vi "Calibration Utility.vi"() -> ()   [LabVIEW 2019]
panel:
  in  "Tab 1":enum32{"Page 1", "Page 2"}(tab)
  in  "Main Tab":T1(tab)
  in  "Tab 2":enum32{"Page 1", "Page 2"}(tab)
  out "Title":string="Calibration Utility, vBETA1"
  out "Date":string="2/21/2012"
  out "Time":string="2:11:48 PM"
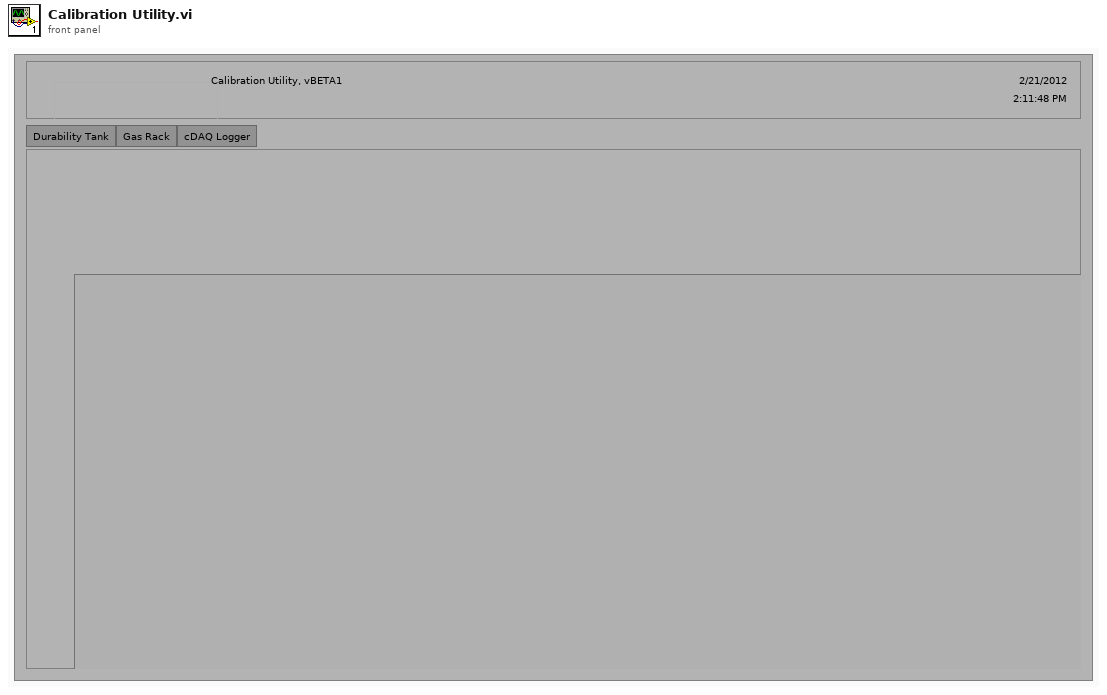
[diagram p1: front panel]
types:
  T1 = enum32{"Netway", "Durability Tank", "Gas Rack", "cDAQ Logger", "Dunk Tank"}
  T2 = cluster{"Error":errorcluster, "OldTab":enum32{"Netway", "Durability Tank", "Gas Rack", "cDAQ Logger", "Dunk Tank"}}
  T3 = enum32{"Page Enabled", "Page Disabled", "Page Disabled & Grayed"}
  T4 = enum32{"Invalid", "Standard", "Closed", "Hidden", "Minimized", "Maximized"}
  T5 = enum32{"invalid app kind", "Development System", "Run Time System", "Student Edition", "Embedded LabVIEW", "Evaluation", "Custom"}
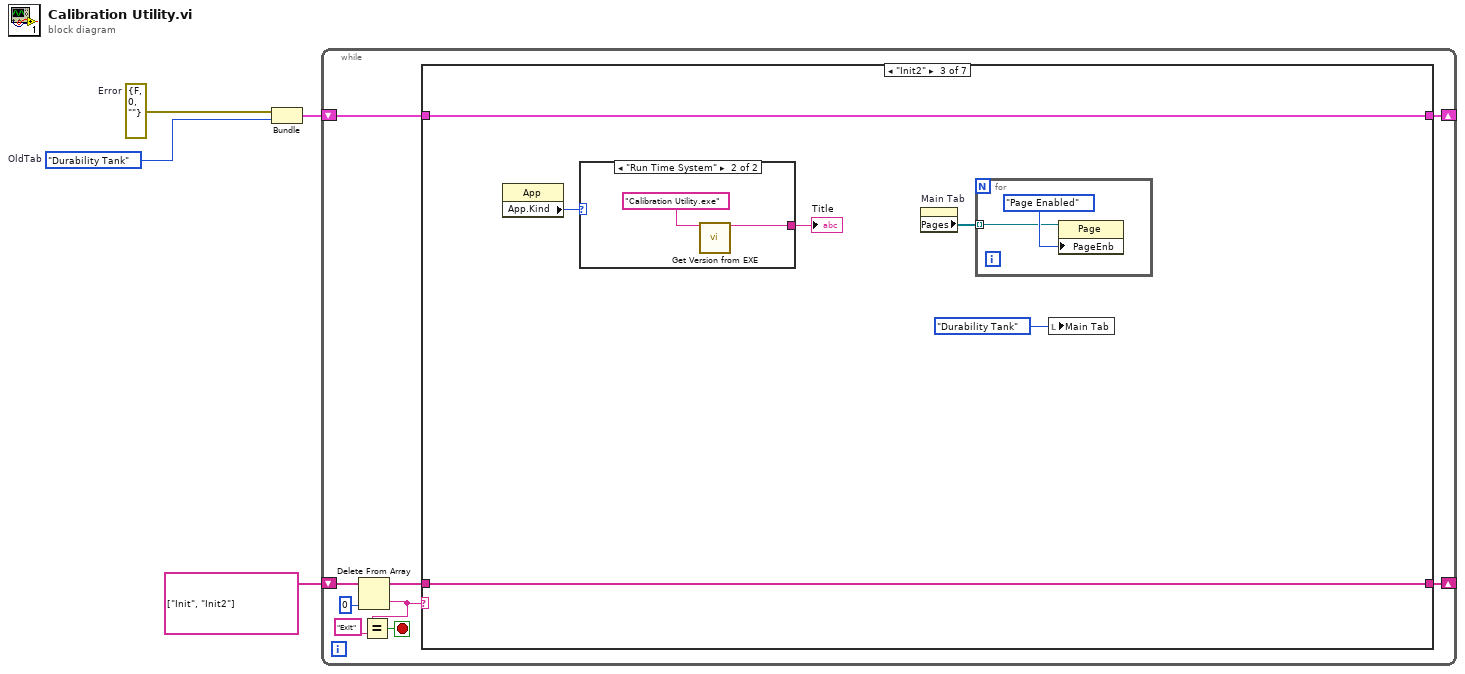
[diagram p0: block diagram]
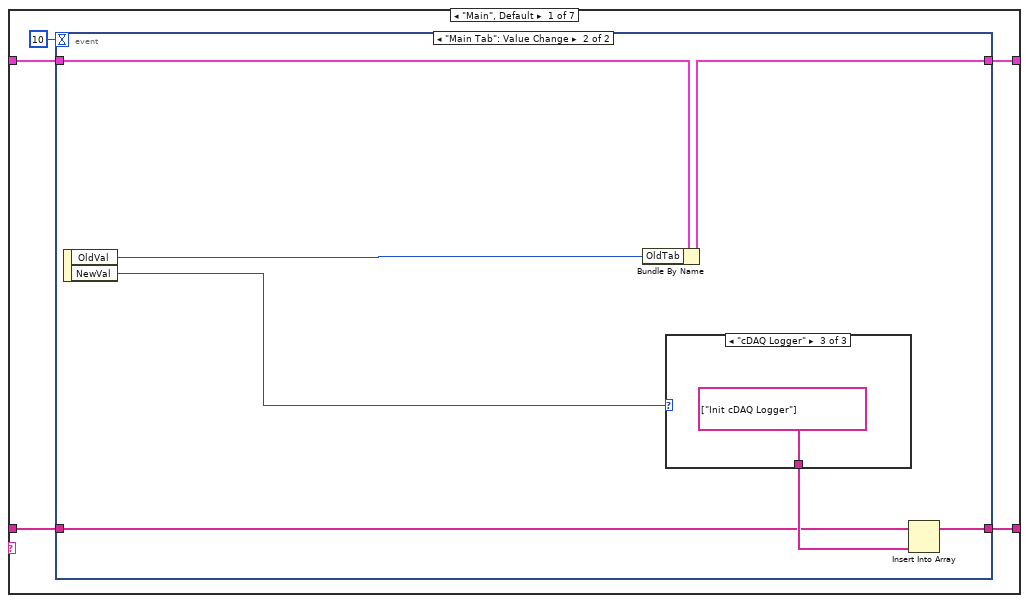
[diagram p2: hidden frame]
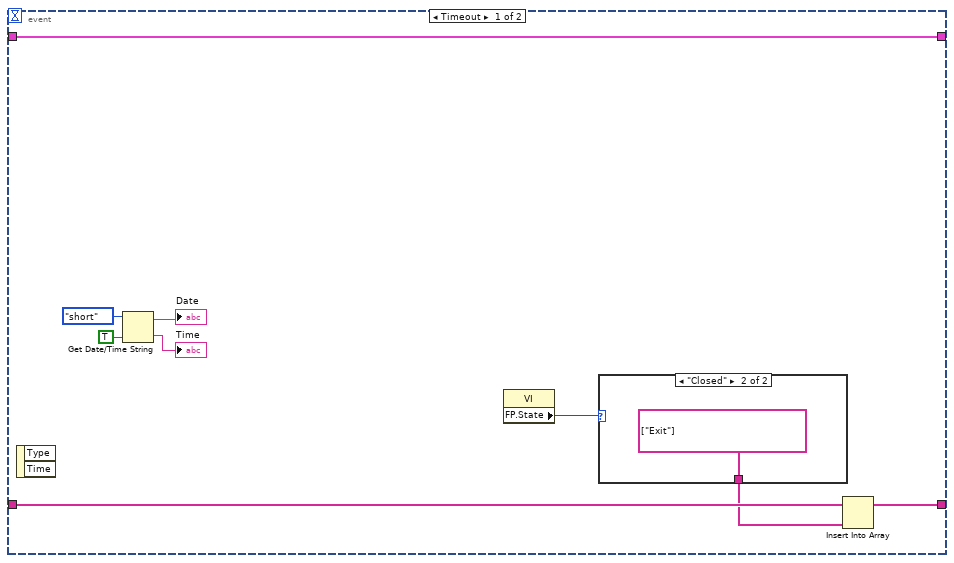
[diagram p3: hidden frame]
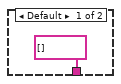
[diagram p4: hidden frame]
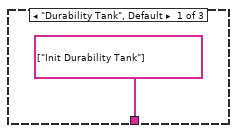
[diagram p5: hidden frame]
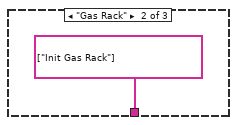
[diagram p6: hidden frame]
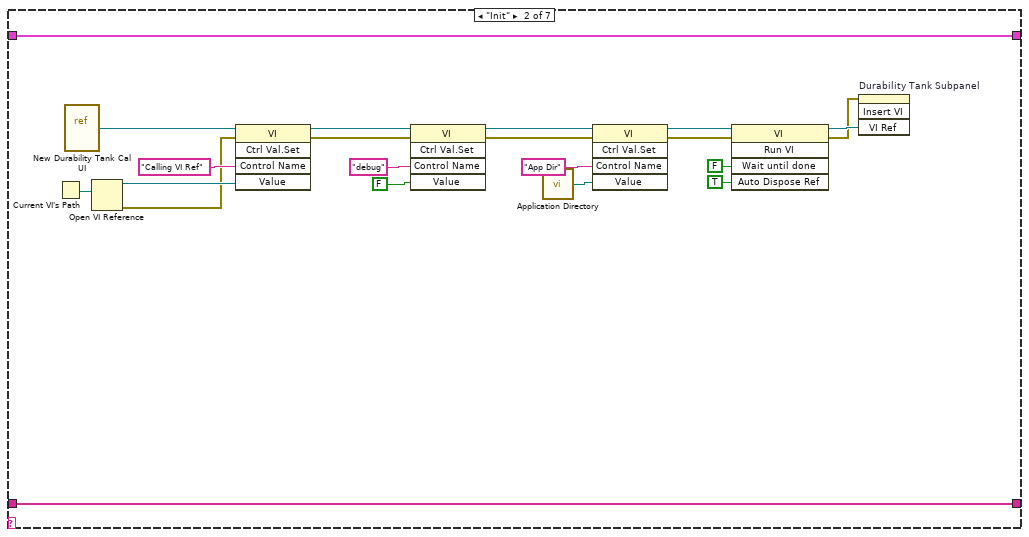
[diagram p7: hidden frame]
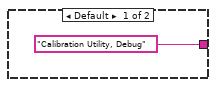
[diagram p8: hidden frame]
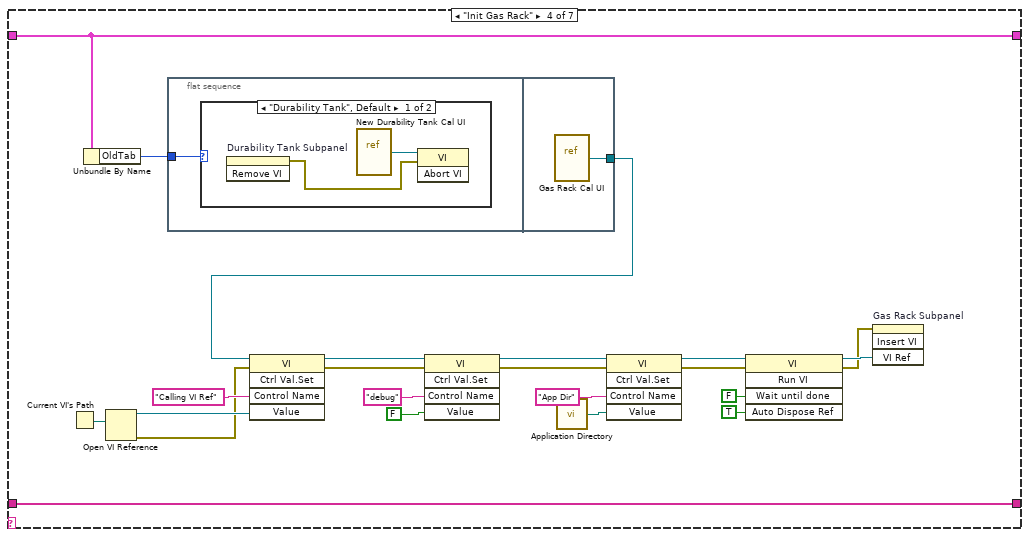
[diagram p9: hidden frame]
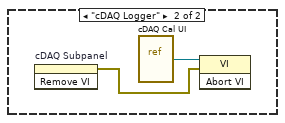
[diagram p10: hidden frame]
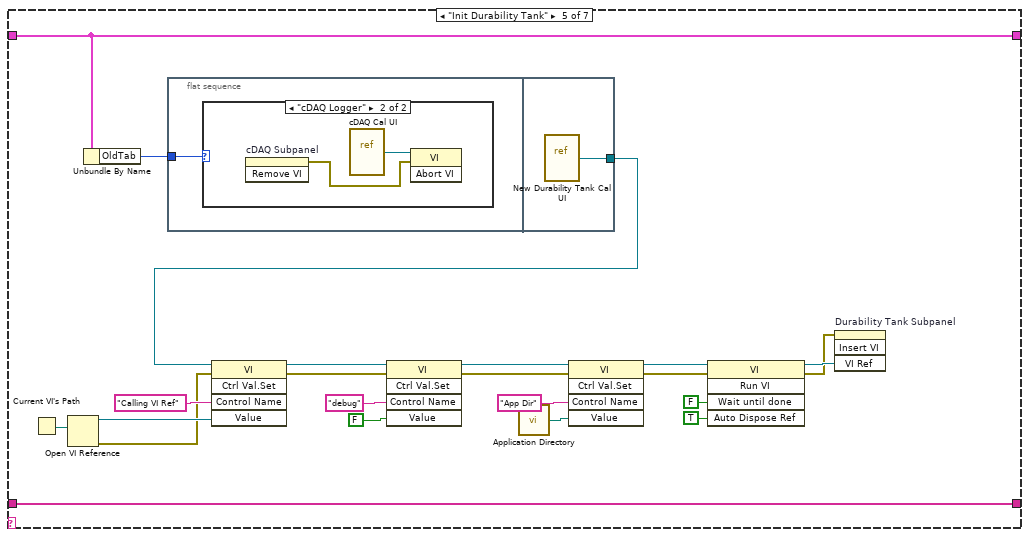
[diagram p11: hidden frame]
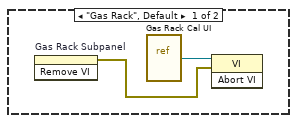
[diagram p12: hidden frame]
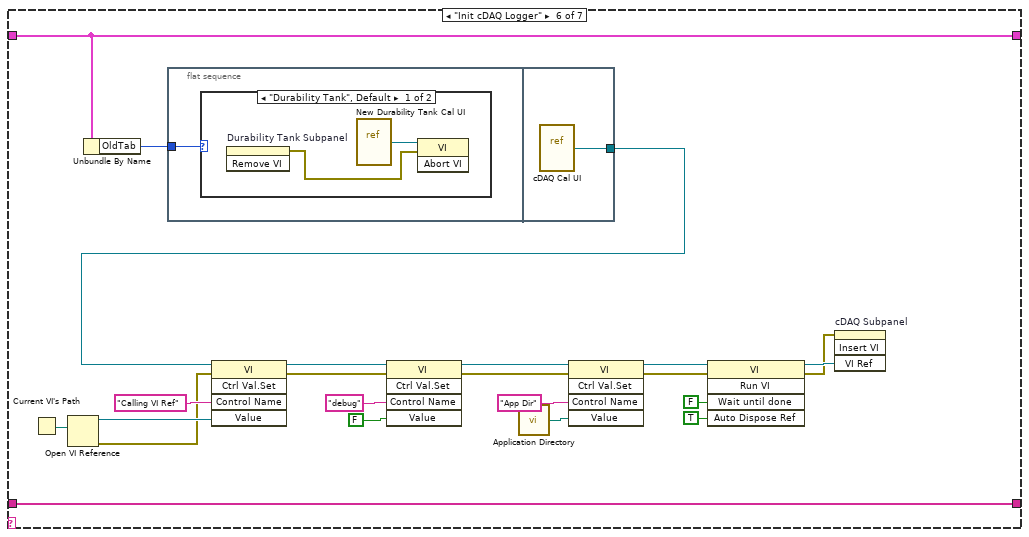
[diagram p13: hidden frame]
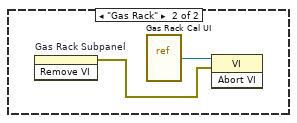
[diagram p14: hidden frame]
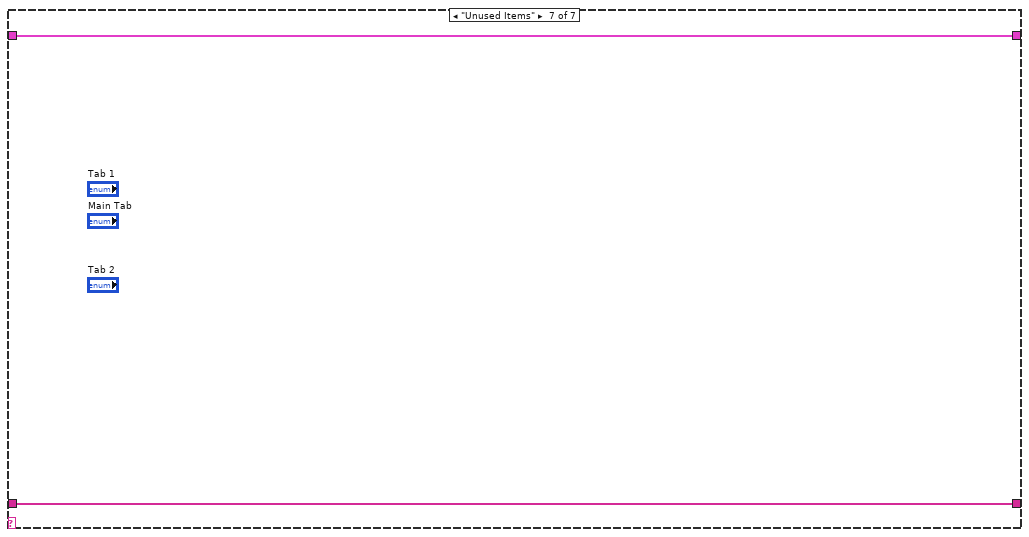
[diagram p15: hidden frame]
diagram:
  w1 = T1."Durability Tank"  # OldTab
  w2 = errorcluster {"status"=FALSE, "code"=0, "source"=""}  # Error
  n1 = Bundle("Error"=w2, "OldTab"=w1) -> (w3:T2)  [unwired: 1 in]
  n2 = while {
    shift-right: [w10] -> _
    shift-left: string[] ["Init", "Init2"] -> [w13]
    shift-right: [w6] -> _
    shift-left: w3 -> [w7]
    stop <- w12 stop-if-true
    n3 = Delete From Array(array=w13, index=0) -> (deleted portion=w9:string, array with subset deleted=w11:string[])  [unwired: 1 in]
    n4 = Equal?(x=w9, y="Exit" ("x")) -> (x = y?=w12:bool)
    n5 = case shown="\"Init2\"" w9 {
      tunnel: [w16 w60 w65 w93 w121 w149 w156] -> w10
      tunnel: w11 -> [w17 w60 w65 w93 w121 w149 w156]
      tunnel: w7 -> [w15 w59 w66 w74 w101 w131 w157]
      tunnel: [w14 w59 w66 w74 w101 w131 w157] -> w6
      frame "Main", Default {
        n6 = event shown="[1] \"Main Tab\": Value Change" {
          selector: _ -> [_ _]
          dyn-events: _ -> [_ _]
          timeout: 10 -> [_ _]
          tunnel: [w22 w35] -> w16
          tunnel: w17 -> [w21 w34]
          tunnel: [w23 w32] -> w14
          tunnel: w15 -> [w23 w33]
          event Timeout {
            n7 = event-data() -> ()  [unwired: 1 in, 2 out]
            n8 = Get Date/Time String(date format (0)=enum16{"short", "long", "abbreviated"}."short", want seconds? (F)=TRUE) -> (date string=→"Date":string, time string=→"Time":string)  [unwired: 1 in]
            n9 = property class="VI"() -> ("FP.State"=w19:T4)  [unwired: 2 in, 2 out]
            n10 = case shown="\"Closed\"" w19 {
              tunnel: [string[] [] string[] ["Exit"]] -> w20
              frame Default {
              }
              frame "Closed" {
              }
            }
            n11 = Insert Into Array(array=w21, new element=w20) -> (w22:string[])  [unwired: 1 in]
          }
          event "Main Tab": Value Change {
            n12 = event-data() -> ("OldVal"=w31:T1, "NewVal"=w30:T1)  [unwired: 1 in]
            n13 = Bundle By Name(cluster=w33, "OldTab"=w31) -> (w32:T2)
            n14 = case shown="\"cDAQ Logger\"" w30 {
              tunnel: [string[] ["Init Durability Tank"] string[] ["Init Gas Rack"] string[] ["Init cDAQ Logger"]] -> w36
              frame "Durability Tank", Default {
              }
              frame "Gas Rack" {
              }
              frame "cDAQ Logger" {
              }
            }
            n15 = Insert Into Array(array=w34, new element=w36) -> (w35:string[])  [unwired: 1 in]
          }
        }
      }
      frame "Init" {
        n16 = Current VI's Path() -> (path=w55:path)
        n17 = vi-ref "New Durability Tank Cal UI.vi"() -> (w54:refnum<vi>)
        n18 = Open VI Reference(vi path=w55) -> (vi reference=w49:refnum<vi>, error out=w40:errorcluster)  [unwired: 5 in]
        n19 = invoke class="VI" method="Ctrl Val.Set"(reference=w54, error in=w40, "Control Name"="Calling VI Ref", "Value"=w49) -> (reference out=w53:refnum<vi>, error out=w44:errorcluster)  [unwired: 1 in, 3 out]
        n20 = invoke class="VI" method="Ctrl Val.Set"(reference=w53, error in=w44, "Control Name"="debug", "Value"=FALSE ("Wait Until Done")) -> (reference out=w52:refnum<vi>, error out=w43:errorcluster)  [unwired: 1 in, 3 out]
        n21 = call <vilib>:"Application Directory.vi"() -> ("Application Directory"=w45:path)
        n22 = invoke class="VI" method="Ctrl Val.Set"(reference=w52, error in=w43, "Control Name"="App Dir", "Value"=w45) -> (reference out=w51:refnum<vi>, error out=w42:errorcluster)  [unwired: 1 in, 3 out]
        n23 = invoke class="VI" method="Run VI"(reference=w51, error in=w42, "Wait until done"=FALSE ("Wait Until Done"), "Auto Dispose Ref"=TRUE ("Auto Dispose Reference")) -> (reference out=w56:refnum<vi>, error out=w41:errorcluster)  [unwired: 1 in, 3 out]
        n24 = invoke on="Durability Tank Subpanel" class="SubPnl" method="Insert VI"(error in=w41, "VI Ref"=w56) -> ()  [unwired: 2 in, 4 out]
      }
      frame "Init2" {
        n25 = property class="App"() -> ("App.Kind"=w63:T5)  [unwired: 2 in, 2 out]
        n26 = case shown="\"Run Time System\"" w63 {
          tunnel: ["Calibration Utility, Debug" ("Name and Version") w69] -> w62
          frame Default {
          }
          frame "Run Time System" {
            n27 = call "Get Version from EXE.vi"("EXE Name"="Calibration Utility.exe") -> ("Name and Version"=w69:string)  [unwired: 12 in, 2 out]
          }
        }
        "Title" <- w62
        n28 = property on="Main Tab" class="TabCtl (strict)"() -> ("Pages"=w64:refnum<vi>[])  [unwired: 2 in, 2 out]
        n29 = for {
          tunnel: w64 -> [w70] mode=indexing
          n30 = property class="Page"(reference=w70, "PageEnb"=T3."Page Enabled" ("Page Enabled State")) -> ()  [unwired: 1 in, 2 out]
        }
        n31 = local write "Main Tab"(T1."Durability Tank" ("Main Tab")) -> ()
      }
      frame "Init Gas Rack" {
        n32 = Current VI's Path() -> (path=w83:path)
        n33 = Unbundle By Name(w74) -> ("OldTab"=w73:T1)
        n34 = Open VI Reference(vi path=w83) -> (vi reference=w88:refnum<vi>, error out=w75:errorcluster)  [unwired: 5 in]
        n35 = flat-sequence {
          tunnel: w73 -> [w94]
          tunnel: [w99] -> w72
          frame #0 {
            n36 = case shown="\"Durability Tank\", Default" w94 {
              frame "Durability Tank", Default {
                n37 = invoke on="Durability Tank Subpanel" class="SubPnl" method="Remove VI"() -> (error out=w95:errorcluster)  [unwired: 3 in, 2 out]
                n38 = vi-ref "New Durability Tank Cal UI.vi"() -> (w96:refnum<vi>)
                n39 = invoke class="VI" method="Abort VI"(reference=w96, error in=w95) -> ()  [unwired: 1 in, 3 out]
              }
              frame "cDAQ Logger" {
                n40 = invoke on="cDAQ Subpanel" class="SubPnl" method="Remove VI"() -> (error out=w97:errorcluster)  [unwired: 3 in, 2 out]
                n41 = vi-ref "cDAQ Cal UI.vi"() -> (w98:refnum<vi>)
                n42 = invoke class="VI" method="Abort VI"(reference=w98, error in=w97) -> ()  [unwired: 1 in, 3 out]
              }
            }
          }
          frame #1 {
            n43 = vi-ref "Gas Rack Cal UI.vi"() -> (w99:refnum<vi>)
          }
        }
        n44 = invoke class="VI" method="Ctrl Val.Set"(reference=w72, error in=w75, "Control Name"="Calling VI Ref", "Value"=w88) -> (reference out=w84:refnum<vi>, error out=w79:errorcluster)  [unwired: 1 in, 3 out]
        n45 = invoke class="VI" method="Ctrl Val.Set"(reference=w84, error in=w79, "Control Name"="debug", "Value"=FALSE ("Wait Until Done")) -> (reference out=w85:refnum<vi>, error out=w78:errorcluster)  [unwired: 1 in, 3 out]
        n46 = call <vilib>:"Application Directory.vi"() -> ("Application Directory"=w92:path)
        n47 = invoke class="VI" method="Ctrl Val.Set"(reference=w85, error in=w78, "Control Name"="App Dir", "Value"=w92) -> (reference out=w86:refnum<vi>, error out=w77:errorcluster)  [unwired: 1 in, 3 out]
        n48 = invoke class="VI" method="Run VI"(reference=w86, error in=w77, "Wait until done"=FALSE ("Wait Until Done"), "Auto Dispose Ref"=TRUE ("Auto Dispose Reference")) -> (reference out=w80:refnum<vi>, error out=w76:errorcluster)  [unwired: 1 in, 3 out]
        n49 = invoke on="Gas Rack Subpanel" class="SubPnl" method="Insert VI"(error in=w76, "VI Ref"=w80) -> ()  [unwired: 2 in, 4 out]
      }
      frame "Init Durability Tank" {
        n50 = Current VI's Path() -> (path=w117:path)
        n51 = Open VI Reference(vi path=w117) -> (vi reference=w112:refnum<vi>, error out=w103:errorcluster)  [unwired: 5 in]
        n52 = Unbundle By Name(w101) -> ("OldTab"=w102:T1)
        n53 = flat-sequence {
          tunnel: w102 -> [w122]
          tunnel: [w127] -> w100
          frame #0 {
            n54 = case shown="\"cDAQ Logger\"" w122 {
              frame "Gas Rack", Default {
                n55 = invoke on="Gas Rack Subpanel" class="SubPnl" method="Remove VI"() -> (error out=w123:errorcluster)  [unwired: 3 in, 2 out]
                n56 = vi-ref "Gas Rack Cal UI.vi"() -> (w124:refnum<vi>)
                n57 = invoke class="VI" method="Abort VI"(reference=w124, error in=w123) -> ()  [unwired: 1 in, 3 out]
              }
              frame "cDAQ Logger" {
                n58 = invoke on="cDAQ Subpanel" class="SubPnl" method="Remove VI"() -> (error out=w125:errorcluster)  [unwired: 3 in, 2 out]
                n59 = vi-ref "cDAQ Cal UI.vi"() -> (w126:refnum<vi>)
                n60 = invoke class="VI" method="Abort VI"(reference=w126, error in=w125) -> ()  [unwired: 1 in, 3 out]
              }
            }
          }
          frame #1 {
            n61 = vi-ref "New Durability Tank Cal UI.vi"() -> (w127:refnum<vi>)
          }
        }
        n62 = invoke class="VI" method="Ctrl Val.Set"(reference=w100, error in=w103, "Control Name"="Calling VI Ref", "Value"=w112) -> (reference out=w116:refnum<vi>, error out=w107:errorcluster)  [unwired: 1 in, 3 out]
        n63 = invoke class="VI" method="Ctrl Val.Set"(reference=w116, error in=w107, "Control Name"="debug", "Value"=FALSE ("Wait Until Done")) -> (reference out=w115:refnum<vi>, error out=w106:errorcluster)  [unwired: 1 in, 3 out]
        n64 = call <vilib>:"Application Directory.vi"() -> ("Application Directory"=w108:path)
        n65 = invoke class="VI" method="Ctrl Val.Set"(reference=w115, error in=w106, "Control Name"="App Dir", "Value"=w108) -> (reference out=w114:refnum<vi>, error out=w105:errorcluster)  [unwired: 1 in, 3 out]
        n66 = invoke class="VI" method="Run VI"(reference=w114, error in=w105, "Wait until done"=FALSE ("Wait Until Done"), "Auto Dispose Ref"=TRUE ("Auto Dispose Reference")) -> (reference out=w118:refnum<vi>, error out=w104:errorcluster)  [unwired: 1 in, 3 out]
        n67 = invoke on="Durability Tank Subpanel" class="SubPnl" method="Insert VI"(error in=w104, "VI Ref"=w118) -> ()  [unwired: 2 in, 4 out]
      }
      frame "Init cDAQ Logger" {
        n68 = Current VI's Path() -> (path=w146:path)
        n69 = Open VI Reference(vi path=w146) -> (vi reference=w141:refnum<vi>, error out=w133:errorcluster)  [unwired: 5 in]
        n70 = Unbundle By Name(w131) -> ("OldTab"=w132:T1)
        n71 = flat-sequence {
          tunnel: w132 -> [w150]
          tunnel: [w155] -> w130
          frame #0 {
            n72 = case shown="\"Durability Tank\", Default" w150 {
              frame "Durability Tank", Default {
                n73 = invoke on="Durability Tank Subpanel" class="SubPnl" method="Remove VI"() -> (error out=w151:errorcluster)  [unwired: 3 in, 2 out]
                n74 = vi-ref "New Durability Tank Cal UI.vi"() -> (w152:refnum<vi>)
                n75 = invoke class="VI" method="Abort VI"(reference=w152, error in=w151) -> ()  [unwired: 1 in, 3 out]
              }
              frame "Gas Rack" {
                n76 = invoke on="Gas Rack Subpanel" class="SubPnl" method="Remove VI"() -> (error out=w153:errorcluster)  [unwired: 3 in, 2 out]
                n77 = vi-ref "Gas Rack Cal UI.vi"() -> (w154:refnum<vi>)
                n78 = invoke class="VI" method="Abort VI"(reference=w154, error in=w153) -> ()  [unwired: 1 in, 3 out]
              }
            }
          }
          frame #1 {
            n79 = vi-ref "cDAQ Cal UI.vi"() -> (w155:refnum<vi>)
          }
        }
        n80 = invoke class="VI" method="Ctrl Val.Set"(reference=w130, error in=w133, "Control Name"="Calling VI Ref", "Value"=w141) -> (reference out=w145:refnum<vi>, error out=w136:errorcluster)  [unwired: 1 in, 3 out]
        n81 = invoke class="VI" method="Ctrl Val.Set"(reference=w145, error in=w136, "Control Name"="debug", "Value"=FALSE ("Wait Until Done")) -> (reference out=w144:refnum<vi>, error out=w135:errorcluster)  [unwired: 1 in, 3 out]
        n82 = call <vilib>:"Application Directory.vi"() -> ("Application Directory"=w137:path)
        n83 = invoke class="VI" method="Ctrl Val.Set"(reference=w144, error in=w135, "Control Name"="App Dir", "Value"=w137) -> (reference out=w143:refnum<vi>, error out=w134:errorcluster)  [unwired: 1 in, 3 out]
        n84 = invoke class="VI" method="Run VI"(reference=w143, error in=w134, "Wait until done"=FALSE ("Wait Until Done"), "Auto Dispose Ref"=TRUE ("Auto Dispose Reference")) -> (reference out=w129:refnum<vi>, error out=w128:errorcluster)  [unwired: 1 in, 3 out]
        n85 = invoke on="cDAQ Subpanel" class="SubPnl" method="Insert VI"(error in=w128, "VI Ref"=w129) -> ()  [unwired: 2 in, 4 out]
      }
      frame "Unused Items" {
      }
    }
  }
